vi "Check Cricket.vi"(7 "Packed refs":T1, 8 "error in (no error)":errorcluster, 11 "Board Game in":refnum<class "Board Game.lvclass">) -> (0 "error out":errorcluster, 3 "Board Game out":refnum<class "Board Game.lvclass">)   [LabVIEW 2021, in "Board Game.lvclass"]
uses:
  Board Game.lvclass
  Application/Packed Refs.ctl
  GameEl_class/private/Enum Direction.ctl
  Board Game.lvclass/Board Game.ctl
  GameEl_class/GameEl.lvclass/GameEl.ctl
  Imposible_Snake_v2/LVApp/Modules/Sound Manager/Typedefs/Sound Effects.ctl
  Cricket/Cricket.lvclass/Cricket.ctl
  <vilib>/numeric/Random Number (Range) U64.vi
  GameEl_class/Write Visible.vi
  Cricket/Write Init Cricket.vi
  Snake_class/Read Snake Head.vi
  GameEl_class/Read Visible.vi
  GameEl_class/Read position.vi
  <vilib>/numeric/sub_Random U32.vi
  Cricket/Cricket.lvclass
  C:/Users/poche/Programs/LabVIEW/imposible snake/GameEl_class/GameEl.lvclass
  Snake_class/Snake.lvclass
  Imposible_Snake_v2/LVApp/Modules/Sound Manager/Sound Manager.lvlib
  GameEl_class/GameEl.lvclass
  Application/Game.lvclass
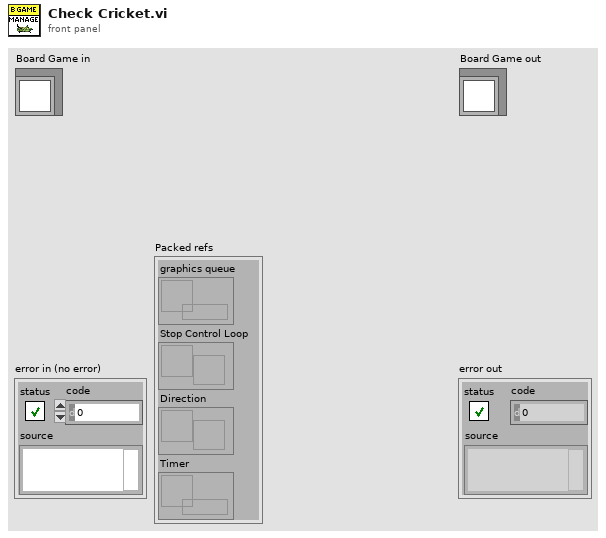
[diagram p1: front panel]
types:
  T1 = typedef "Game.lvclass/Packed Refs.ctl" = cluster{"graphics queue":refnum<queue>, "Stop Control Loop":refnum<user-event>, "Direction":refnum<notifier>, "Timer":refnum<data-value>}
  T2 = typedef "Sound Manager.lvlib/Sound Effects.ctl" = enum16{"Bomb In", "Bomb Out", "Bomb Touched", "Game Over", "Victory", "Eat", "10 Fruits", "Eat2", "Eat3", "Eat4", "MaxShield", "Shield", "10p", "Grape In", "Grape Out", "20p", "30p", "40p", "50p", "60p", "70p", "80p", "90p", "100p", "All shields cracked", "Mouse In", "Mouse Out", "Mouse Eaten", "Grape Eaten", "States Recover", "Broken Shield", "Bonus", "Happy Time", "explode", "Game over musica", "Back Music", "Shield Catch", "Evil lough", "Cricket In", "Cricket eaten", "Lets Go", "Jump1", "Jump2", "Jump3", "Unstoppable", "Troll Music", "winner", "menu"}
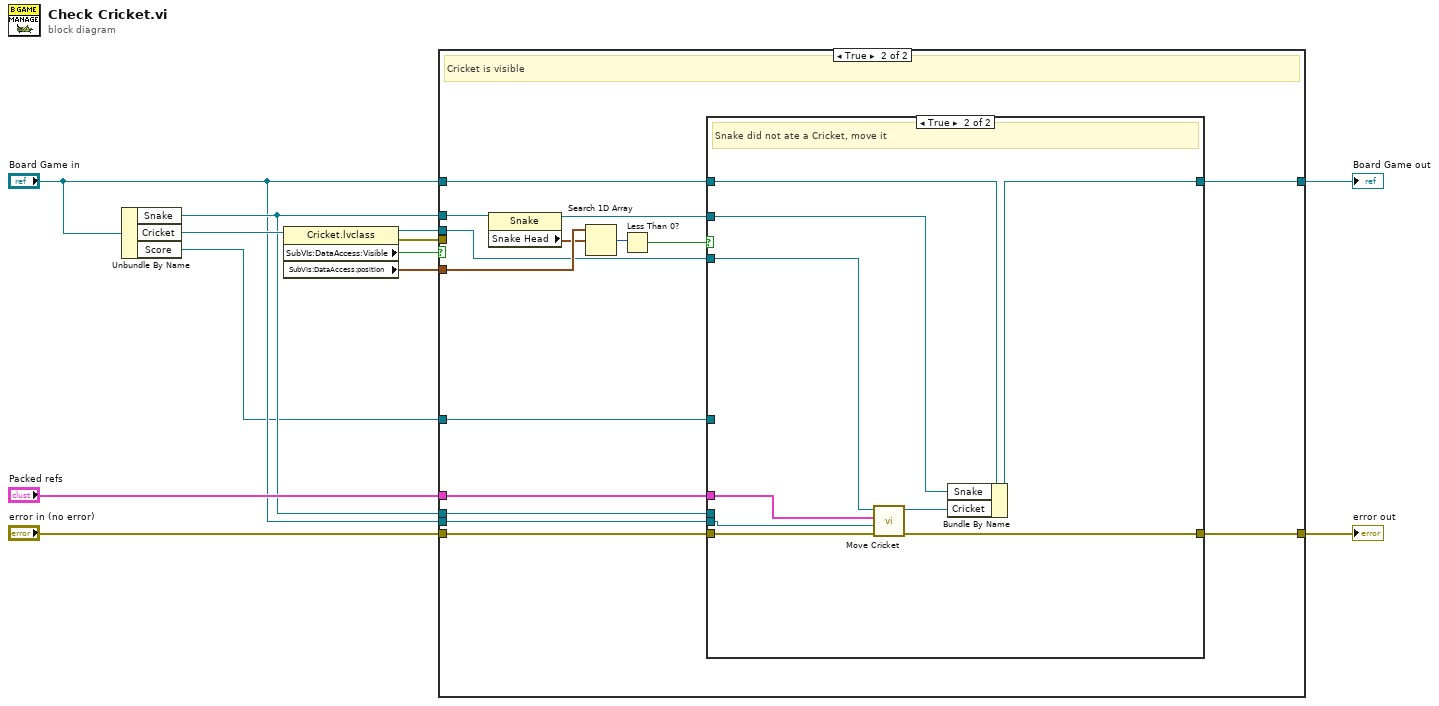
[diagram p0: block diagram]
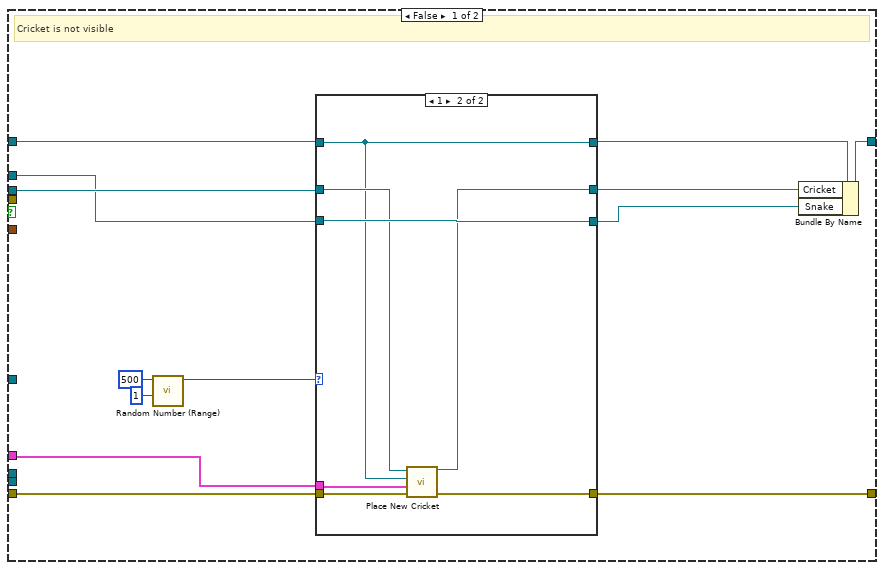
[diagram p2: hidden frame]
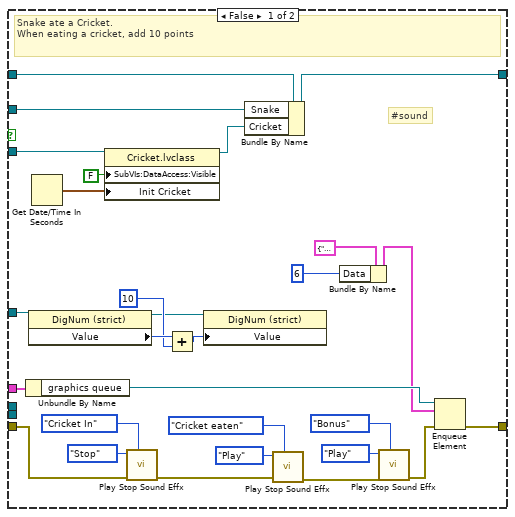
[diagram p4: hidden frame]
diagram:
  n1 = Unbundle By Name("Board Game in") -> ("Snake"=w4:refnum<class "Snake.lvclass">, "Cricket"=w12:refnum<class "Cricket.lvclass">, "Score"=w2:refnum<vi>)
  n2 = property class="Cricket.lvclass"(reference=w12) -> (reference out=w9:refnum<class "Cricket.lvclass">, error out=w7:errorcluster, "SubVIs:DataAccess:Visible"=w10:bool, "SubVIs:DataAccess:position"=w8:cluster{"x":dbl, "y":dbl}[])  [unwired: 1 in]
  n3 = case shown="True" w10 {
    tunnel: "error in (no error)" -> [w23 w48]
    tunnel: "Board Game in" -> [w25 w46]
    tunnel: [w20 w45] -> w6
    tunnel: [w22 w47] -> w1
    tunnel: w9 -> [w21 w38]
    tunnel: w4 -> [w15 w37]
    tunnel: w8 -> [_ w51]
    tunnel: w7 -> [_ _]
    tunnel: "Packed refs" -> [w14 w42]
    tunnel: w4 -> [_ w41]
    tunnel: "Board Game in" -> [_ w40]
    tunnel: w2 -> [_ w39]
    frame False {
      # "Cricket is not visible"
      n4 = call-poly <vilib>:"Random Number (Range).vi"("lower bound (0)"=u64 1, "upper bound (100)"=u64 500) -> ("number"=w13:u64)  [unwired: 9 in]
      n5 = case shown="1" w13 {
        tunnel: w25 -> [w29 w30]
        tunnel: [w29 w30] -> w24
        tunnel: w23 -> [w28 w31]
        tunnel: [w28 w34] -> w22
        tunnel: w21 -> [w27 w33]
        tunnel: [w27 w35] -> w19
        tunnel: w15 -> [w26 w36]
        tunnel: [w26 w36] -> w18
        tunnel: w14 -> [_ w32]
        frame 0, Default {
        }
        frame 1 {
          n6 = call "Place New Cricket.vi"("error in (no error)"=w31, "Packed refs"=w32, "Board Game in"=w30, "Cricket in"=w33) -> ("error out"=w34:errorcluster, "Cricket out"=w35:refnum<class "Cricket.lvclass">)  [unwired: 5 in, 1 out]
        }
      }
      n7 = Bundle By Name(cluster=w24, "Cricket"=w19, "Snake"=w18) -> (w20:refnum<class "Board Game.lvclass">)
    }
    frame True {
      # "Cricket is visible"
      n8 = property class="Snake"(reference=w37) -> (reference out=w43:refnum<class "Snake.lvclass">, "Snake Head"=w50:cluster{"x":dbl, "y":dbl})  [unwired: 1 in, 1 out]
      n9 = Search 1D Array(1D array=w51, element=w50) -> (index of element=w49:i32)  [unwired: 1 in]
      n10 = Less Than 0?(x=w49) -> (x < 0?=w44:bool)
      n11 = case shown="True" w44 {
        tunnel: w48 -> [w55 w85]
        tunnel: [w70 w84] -> w47
        tunnel: w46 -> [w79 w88]
        tunnel: [w78 w87] -> w45
        tunnel: w38 -> [w77 w82]
        tunnel: w43 -> [w74 w86]
        tunnel: w42 -> [w72 w80]
        tunnel: w41 -> [_ _]
        tunnel: w40 -> [_ w81]
        tunnel: w39 -> [w73 _]
        frame False {
          # "#sound"
          # "Snake ate a Cricket. \nWhen eating a cricket, add 10 points"
          n12 = Unbundle By Name(w72) -> ("graphics queue"=w65:refnum<queue>)
          n13 = property class="DigNum (strict)"(reference=w73) -> (reference out=w66:refnum<vi>, "Value"=w69:u16)  [unwired: 1 in, 1 out]
          n14 = Get Date/Time In Seconds() -> (seconds since 1Jan1904=w71:timestamp)
          n15 = property class="Cricket.lvclass"(reference=w77, "SubVIs:DataAccess:Visible"=FALSE ("Visible"), "Init Cricket"=w71) -> (reference out=w76:refnum<class "Cricket.lvclass">)  [unwired: 1 in, 1 out]
          n16 = call "Play Stop Sound Effx.vi"("Sound Effect"=Sound_Effects."Cricket In", "Error In"=w55, "Function"=enum16{"Play", "Stop"}."Stop") -> ("error in (no error)"=w54:errorcluster)  [unwired: 8 in]
          n17 = Add(x=w69, y=u16 10) -> (x+y=w67:u16)
          n18 = property class="DigNum (strict)"(reference=w66, "Value"=w67) -> ()  [unwired: 1 in, 2 out]
          n19 = Bundle By Name(cluster=w79, "Snake"=w74, "Cricket"=w76) -> (w78:refnum<class "Board Game.lvclass">)
          n20 = call "Play Stop Sound Effx.vi"("Sound Effect"=Sound_Effects."Cricket eaten", "Error In"=w54, "Function"=enum16{"Play", "Stop"}."Play") -> ("error in (no error)"=w53:errorcluster)  [unwired: 8 in]
          n21 = Bundle By Name(cluster=cluster{"Message":string, "Data":variant} {"Message"="10 Points", "Data"=variant} ("element"), "Data"=u16 6) -> (w63:cluster{"Message":string, "Data":variant})
          n22 = call "Play Stop Sound Effx.vi"("Sound Effect"=Sound_Effects."Bonus", "Error In"=w53, "Function"=enum16{"Play", "Stop"}."Play") -> ("error in (no error)"=w52:errorcluster)  [unwired: 8 in]
          n23 = Enqueue Element(queue=w65, element=w63, error in (no error)=w52) -> (error out=w70:errorcluster)  [unwired: 1 in, 2 out]
        }
        frame True {
          # "Snake did not ate a Cricket, move it"
          n24 = call "Move Cricket.vi"("error in (no error)"=w85, "Board Game in"=w81, "Packed refs"=w80, "Cricket in"=w82) -> ("error out"=w84:errorcluster, "Cricket out"=w83:refnum<class "Cricket.lvclass">)  [unwired: 6 in]
          n25 = Bundle By Name(cluster=w88, "Snake"=w86, "Cricket"=w83) -> (w87:refnum<class "Board Game.lvclass">)
        }
      }
    }
  }
  "error out" <- w1
  "Board Game out" <- w6
